vi "Unit Test - Is CSM Modules.vi"() -> (3 "output cluster":cluster{"VI":bool[], "WhileLoop":bool[]})   [LabVIEW 2017, in "testcase-csmhelper.lvclass"]
uses:
  testcase-csmhelper.lvclass
  <vilib>/Utility/traverseref.llb/TRef TravTarget.ctl
panel:
  out "WhileLoop":bool[](array[boolean])
  out "VI":bool[](array[boolean])
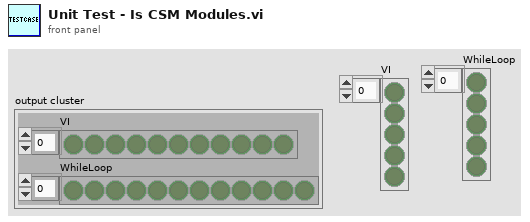
[diagram p1: front panel]
types:
  T1 = typedef "TRef TravTarget.ctl" = enum16{"FP", "BD", "Other"}
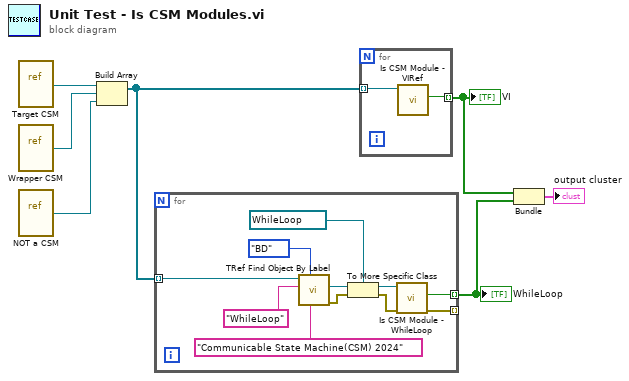
[diagram p0: block diagram]
diagram:
  n1 = vi-ref "Target CSM.vi"() -> (w5:refnum<vi>)
  n2 = vi-ref "Wrapper CSM.vi"() -> (w7:refnum<vi>)
  n3 = vi-ref "NOT a CSM.vi"() -> (w6:refnum<vi>)
  n4 = Build Array(w5, w7, w6) -> (w4:refnum<vi>[])
  n5 = for {
    tunnel: w4 -> [w18] mode=indexing
    tunnel: [w12] -> w2 mode=indexing
    tunnel: [w9] -> _ mode=indexing
    n6 = call <vilib>:"TRef Find Object By Label.vi"("Label"="Communicable State Machine(CSM) 2024", "Traverse Target"=TRef_TravTarget."BD", "Class Name"="WhileLoop", "VI Ref"=w18) -> ("error out"=w11:errorcluster, "Found Obj Ref"=w15:refnum<vi>)  [unwired: 4 in, 2 out]
    n7 = To More Specific Class(target class=refnum<vi> refnum ("WhileLoop in"), reference=w15, error in=w11) -> (specific class reference=w14:refnum<vi>, error out=w10:errorcluster)
    n8 = call "Is CSM Module - WhileLoop.vi"("error in (no error)"=w10, "WhileLoop in"=w14) -> ("error out"=w9:errorcluster, "Is CSM Module?"=w12:bool)  [unwired: 7 in, 1 out]
  }
  "WhileLoop" <- w2
  n9 = for {
    tunnel: w4 -> [w20] mode=indexing
    tunnel: [w19] -> w3 mode=indexing
    n10 = call "Is CSM Module - VIRef.vi"("VIRef"=w20) -> ("Is CSM Module?"=w19:bool)  [unwired: 8 in, 2 out]
  }
  "VI" <- w3
  n11 = Bundle(w3, w2) -> (→"output cluster":cluster{bool[], bool[]})  [unwired: 1 in]
